vi "SubVI-SensorManipulation2.vi"(8 "error in":errorcluster, 11 "Array in":dbl[](array[numeric])) -> (0 "error out":errorcluster, 3 "Array out":dbl[](array[numeric]))   [LabVIEW 2021]
panel:
  in  "Temperature Offset":dbl
  in  "Binary 2":bool
  in  "AIN Range":u16(ring) items=["LJ_rgBIP10V", "LJ_rgBIP1V", "LJ_rgBIPP1V", "LJ_rgBIPP01V"]
  in  "FirstFound":bool=TRUE
  in  "Address":string="1"
  out "Error Message 2":string="No Error"
  out "Cold Junction Temp":dbl=41420.0 format="%.6f"
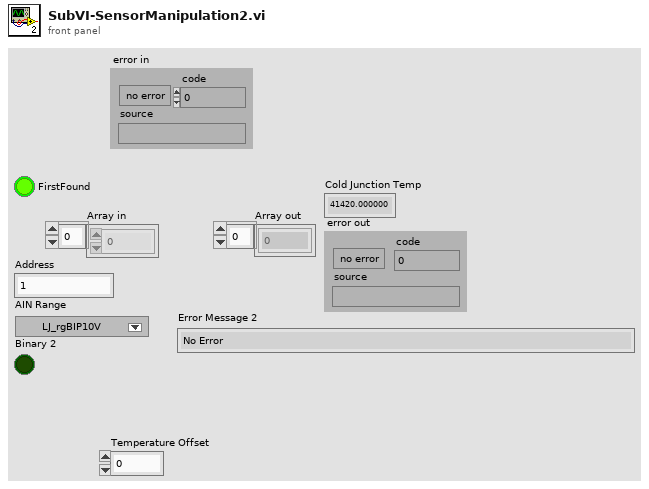
[diagram p1: front panel]
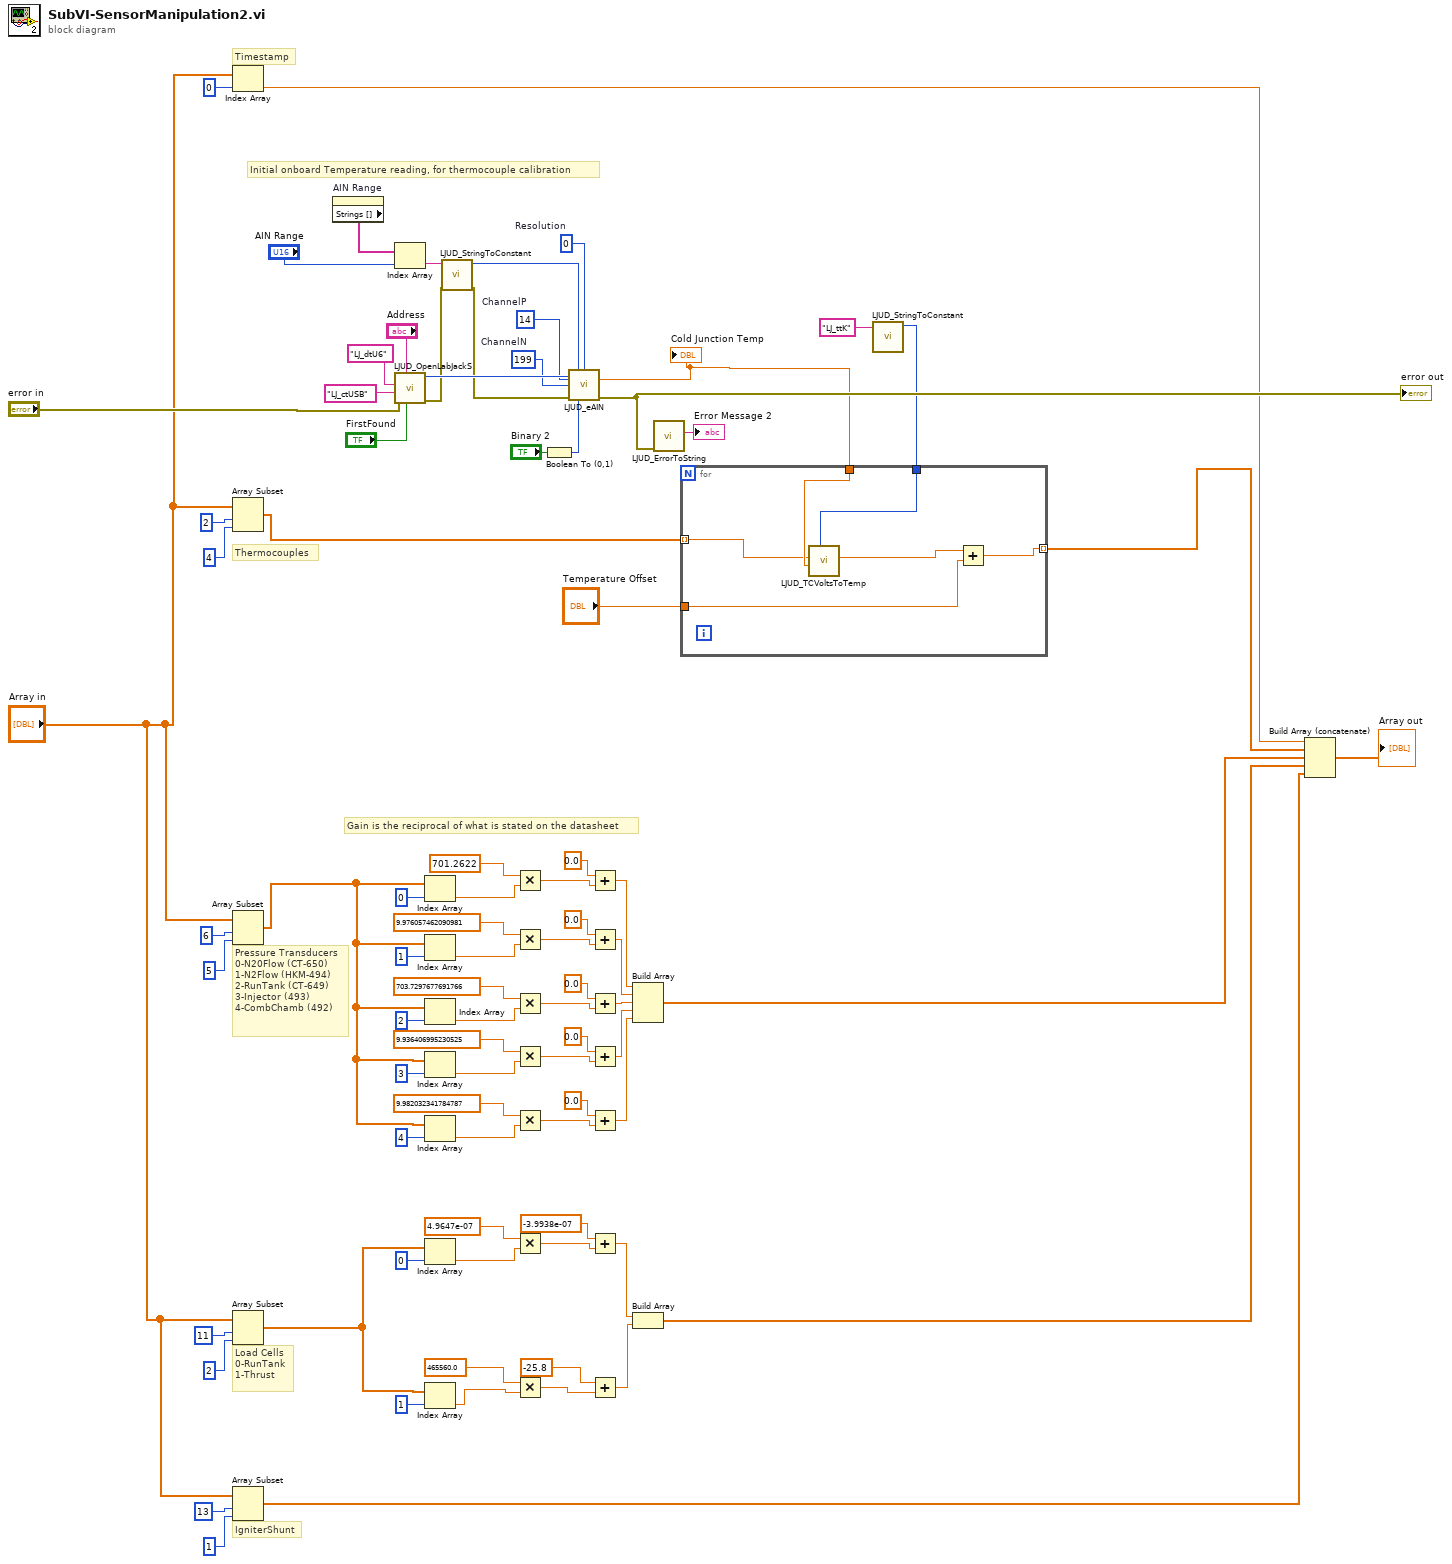
[diagram p0: block diagram]
diagram:
  w74 = 0  # Resolution
  w64 = 199  # ChannelN
  w65 = 14  # ChannelP
  # "Gain is the reciprocal of what is stated on the datasheet"
  # "Timestamp"
  # "IgniterShunt"
  # "Thermocouples"
  # "Pressure Transducers\n0-N20Flow (CT-650)\n1-N2Flow (HKM-494)\n2-RunTank (CT-649)\n3-Injector (493)\n4-CombChamb (492)"
  # "Load Cells\n0-RunTank\n1-Thrust"
  # "Initial onboard Temperature reading, for thermocouple calibration"
  n1 = Index Array(array="Array in", index=0) -> (element=w56:dbl)
  n2 = Array Subset(array="Array in", index=2, length=4) -> (w82:dbl[])
  n3 = Array Subset(array="Array in", index=6, length=5) -> (w11:dbl[])
  n4 = Array Subset(array="Array in", index=11, length=2) -> (w39:dbl[])
  n5 = Array Subset(array="Array in", index=13, length=1) -> (w1:dbl[])
  n6 = property on="AIN Range" class="Ring (strict)"() -> ("Strings []"=w70:string[])  [unwired: 2 in, 2 out]
  n7 = Index Array(array=w70, index="AIN Range") -> (element=w68:string)
  n8 = call "LJUD_OpenLabJackS.vi"("FirstFound"="FirstFound", "Address"="Address", "error in"="error in", "ConnectionType"="LJ_ctUSB", "DeviceType"="LJ_dtU6") -> ("error out"=w73:errorcluster, "Handle"=w77:i32)  [unwired: 4 in, 1 out]
  n9 = Index Array(array=w11, index=0) -> (element=w35:dbl)
  n10 = Index Array(array=w11, index=1) -> (element=w30:dbl)
  n11 = Index Array(array=w11, index=2) -> (element=w25:dbl)
  n12 = Index Array(array=w11, index=3) -> (element=w20:dbl)
  n13 = Index Array(array=w11, index=4) -> (element=w15:dbl)
  n14 = Index Array(array=w39, index=0) -> (element=w49:dbl)
  n15 = Index Array(array=w39, index=1) -> (element=w38:dbl)
  n16 = call "LJUD_StringToConstant.vi"("error in"=w73, "String"=w68) -> ("error out"=w72:errorcluster, "Constant Number"=w75:i32)  [unwired: 8 in]
  n17 = Multiply(x=701.2622, y=w35) -> (x*y=w34:dbl)
  n18 = Multiply(x=9.976057462090981, y=w30) -> (x*y=w29:dbl)
  n19 = Multiply(x=703.7297677691766, y=w25) -> (x*y=w24:dbl)
  n20 = Multiply(x=9.936406995230525, y=w20) -> (x*y=w19:dbl)
  n21 = Multiply(x=9.982032341784787, y=w15) -> (x*y=w14:dbl)
  n22 = Multiply(x=4.9647e-07, y=w49) -> (x*y=w48:dbl)
  n23 = Multiply(x=465560.0, y=w38) -> (x*y=w47:dbl)
  n24 = Boolean To (0,1)(Boolean="Binary 2") -> (0, 1=w66:i16)
  n25 = call "LJUD_eAIN.vi"("Handle In"=w77, "Range"=w75, "Resolution"=w74, "ChannelP"=w65, "ChannelN"=w64, "error in"=w72, "Binary"=w66) -> ("Voltage"=w61:dbl, "error out"=w80:errorcluster)  [unwired: 6 in, 1 out]
  "Cold Junction Temp" <- w61
  "error out" <- w80
  n26 = Add(x=0.0, y=w34) -> (x+y=w10:dbl)
  n27 = Add(x=0.0, y=w29) -> (x+y=w9:dbl)
  n28 = Add(x=0.0, y=w24) -> (x+y=w8:dbl)
  n29 = Add(x=0.0, y=w19) -> (x+y=w7:dbl)
  n30 = Add(x=0.0, y=w14) -> (x+y=w6:dbl)
  n31 = Add(x=-3.9938e-07, y=w48) -> (x+y=w46:dbl)
  n32 = Add(x=-25.8, y=w47) -> (x+y=w45:dbl)
  n33 = Build Array(w10, w9, w8, w7, w6) -> (w5:dbl[])
  n34 = Build Array(w46, w45) -> (w44:dbl[])
  n35 = call "LJUD_ErrorToString.vi"("error in"=w80) -> ("String"=→"Error Message 2":string)  [unwired: 10 in]
  n36 = call "LJUD_StringToConstant.vi"("String"="LJ_ttK") -> ("Constant Number"=w62:i32)  [unwired: 9 in, 1 out]
  n37 = for {
    tunnel: w82 -> [w88] mode=indexing
    tunnel: w62 -> [w90]
    tunnel: w61 -> [w89]
    tunnel: [w85] -> w57 mode=indexing
    tunnel: "Temperature Offset" -> [w87]
    n38 = call "LJUD_TCVoltsToTemp.vi"("TCType"=w90, "CJTempK"=w89, "TCVolts"=w88) -> ("TCTempC"=w86:dbl)  [unwired: 5 in, 3 out]
    n39 = Add(x=w86, y=w87) -> (x+y=w85:dbl)
  }
  n40 = Build Array (concatenate)(w56, w57, w5, w44, w1) -> (→"Array out":dbl[])
